vi "thingspeak (SubVI).vi"(0 "Sensor 1 input":dbl, 1 "Sensor 2 input":dbl, 2 "Sensor 3 input":dbl, 3 "Sensor 4 input":dbl, 7 "Sensor 5 input":dbl, 8 "Sensor 6 input":dbl, 9 "API Key":string="NQ2A5BSQS6NT7G9B") -> ()   [LabVIEW 2015]
uses:
  <vilib>/httpClient/LabVIEWHTTPClient.lvlib
panel:
  out "resulting string":string
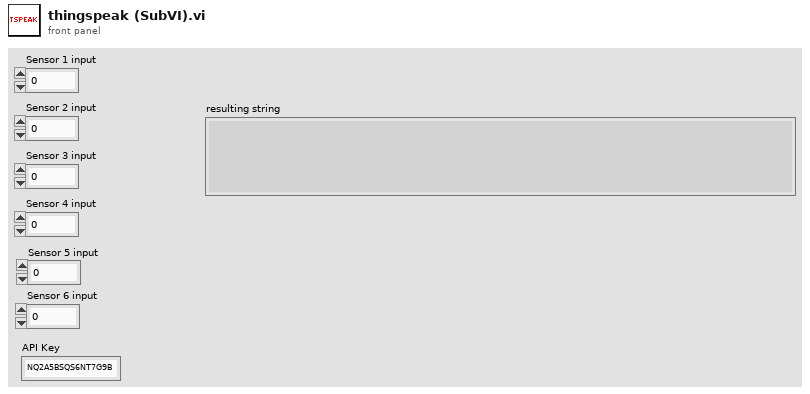
[diagram p1: front panel]
types:
  T1 = typedef "LabVIEWHTTPClient.lvlib/ClientHandle.ctl" = refnum<k1>
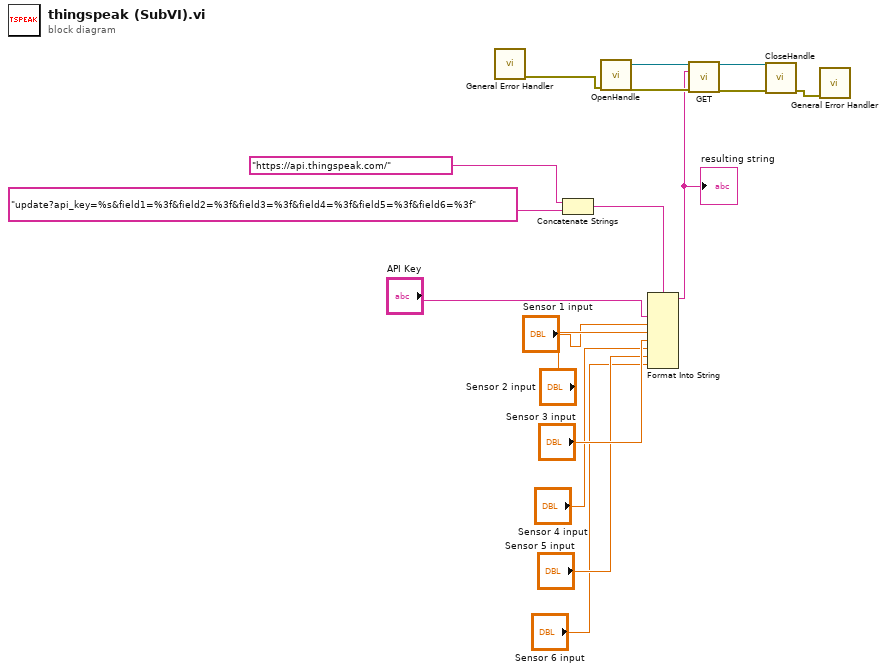
[diagram p0: block diagram]
diagram:
  n1 = call <vilib>:"General Error Handler.vi"() -> ("error out"=w13:errorcluster)  [unwired: 11 in, 4 out]
  n2 = Concatenate Strings("https://api.thingspeak.com/", "update?api_key=%s&field1=%3f&field2=%3f&field3=%3f&field4=%3f&field5=%3f&field6=%3f") -> (w9:string)
  n3 = call <vilib>:"OpenHandle.vi"("error in (no error)"=w13) -> ("client handle out"=w15:T1, "error out"=w10:errorcluster)  [unwired: 13 in]
  n4 = Format Into String(format string=w9, "API Key", "Sensor 1 input", "Sensor 2 input", "Sensor 3 input", "Sensor 4 input", "Sensor 5 input", "Sensor 6 input") -> (resulting string=w8:string)  [unwired: 2 in, 1 out]
  "resulting string" <- w8
  n5 = call <vilib>:"GET.vi"("client handle"=w15, "url"=w8, "error in (no error)"=w10) -> ("client handle out"=w14:T1, "error out"=w11:errorcluster)  [unwired: 9 in, 2 out]
  n6 = call <vilib>:"CloseHandle.vi"("client handle"=w14, "error in (no error)"=w11) -> ("error out"=w12:errorcluster)  [unwired: 13 in]
  n7 = call <vilib>:"General Error Handler.vi"("error in (no error)"=w12) -> ()  [unwired: 10 in, 5 out]
